vi "Find Center.vi"(7 "Tray Number":dbl format="%#_13g", 9 "XYZTheta":dbl[](array[numeric]), 10 "Motion.lvclass":refnum<class "Motion.lvclass">) -> (1 "XYZTheta Centers":dbl[][](array[numeric]), 2 "Motion Out":refnum<class "Motion.lvclass">)   [LabVIEW 2016, in "Assembly Tray.lvclass"]
uses:
  Assembly Tray.lvclass
  Find Tray.ctl
  Controller/Motion/Motion.lvclass
  Controller/Camera/Machine Vision.ctl
  Controller/Camera/Camera.lvclass
panel:
  in  "Machine Vision":T1=enum."Tray Fiducials"
  out "Right Fiducial":dbl[](array[numeric])
  out "Left Fiducial":dbl[](array[numeric])
  out "Gantry":dbl[](array[numeric])
  out "Sum":dbl[](array[numeric])
  out "Camera":dbl[](array[numeric])
  in  "Carrier Tray":T2
  out "Image":T3(plugin-control)
  out "Center":dbl[](array[numeric])
  in  "Position Number":i16
  in  "Go to Center":bool
  in  "Calculate":bool
  in  "Record Bottom":bool
  in  "Record Top":bool
  in  "Go to Bottom Fiducial":bool
  in  "Go to Top Fiducial":bool
  in  "Joystick":bool
  in  "Stop":bool
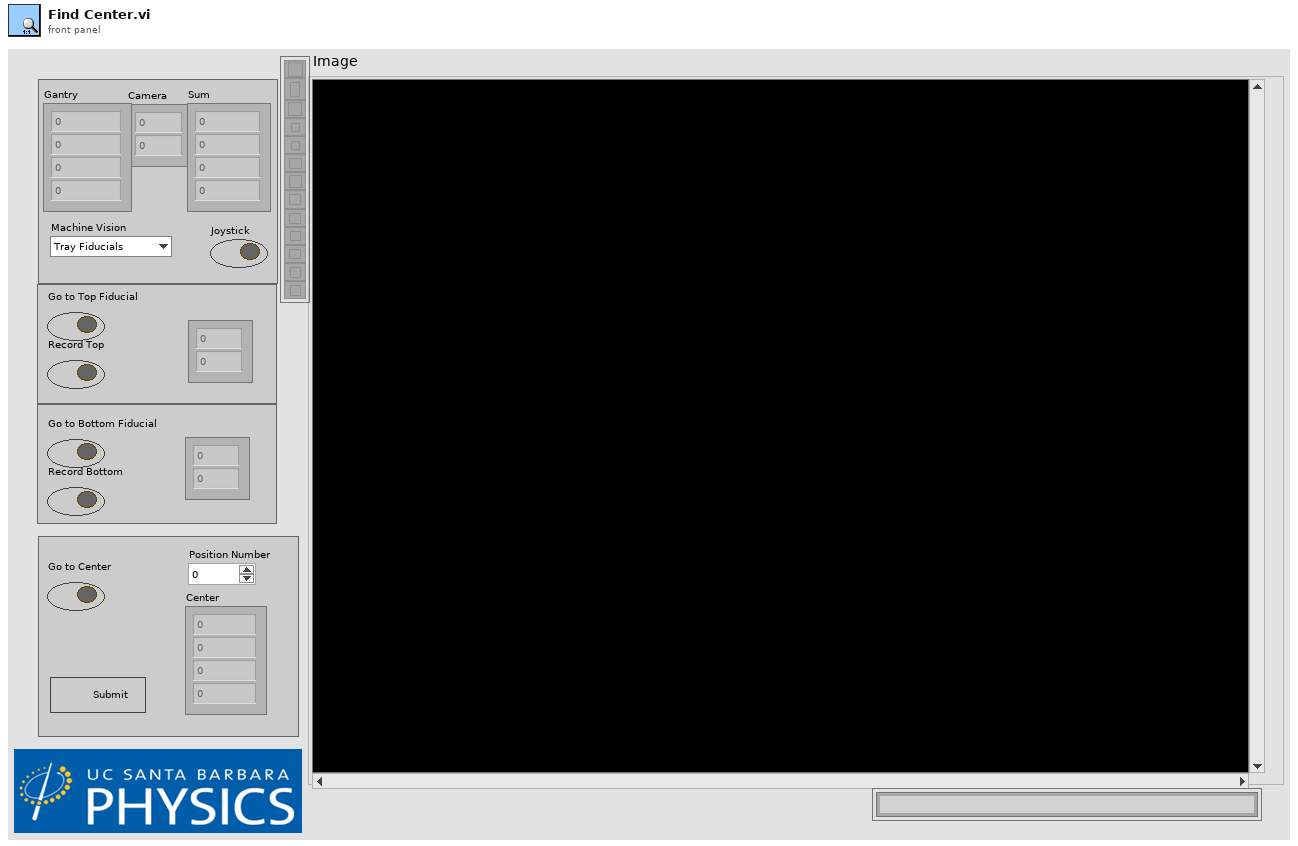
[diagram p1: front panel]
types:
  T1 = typedef "Camera.lvclass/Machine Vision.ctl" = enum16{"None", "Tray Fiducials", "HPK Silicon", "Hexaboard", "Corner (TL, BR)", "Corner (BL, TR)"}
  T2 = typedef "Assembly Tray.lvclass/Find Tray.ctl" = cluster{"Gantry Fiducials":dbl[], "Relative Coordinates":dbl[][], "Camera Fiducials":dbl[][], "XYZTheta Centers":dbl[][], "Workspace Center":dbl[], "Syringe Relative Coordinates":dbl[], "Gantry Region":dbl, "Fiducials":path}
  T3 = typedef "IMAQ Image.ctl" = refnum<image>
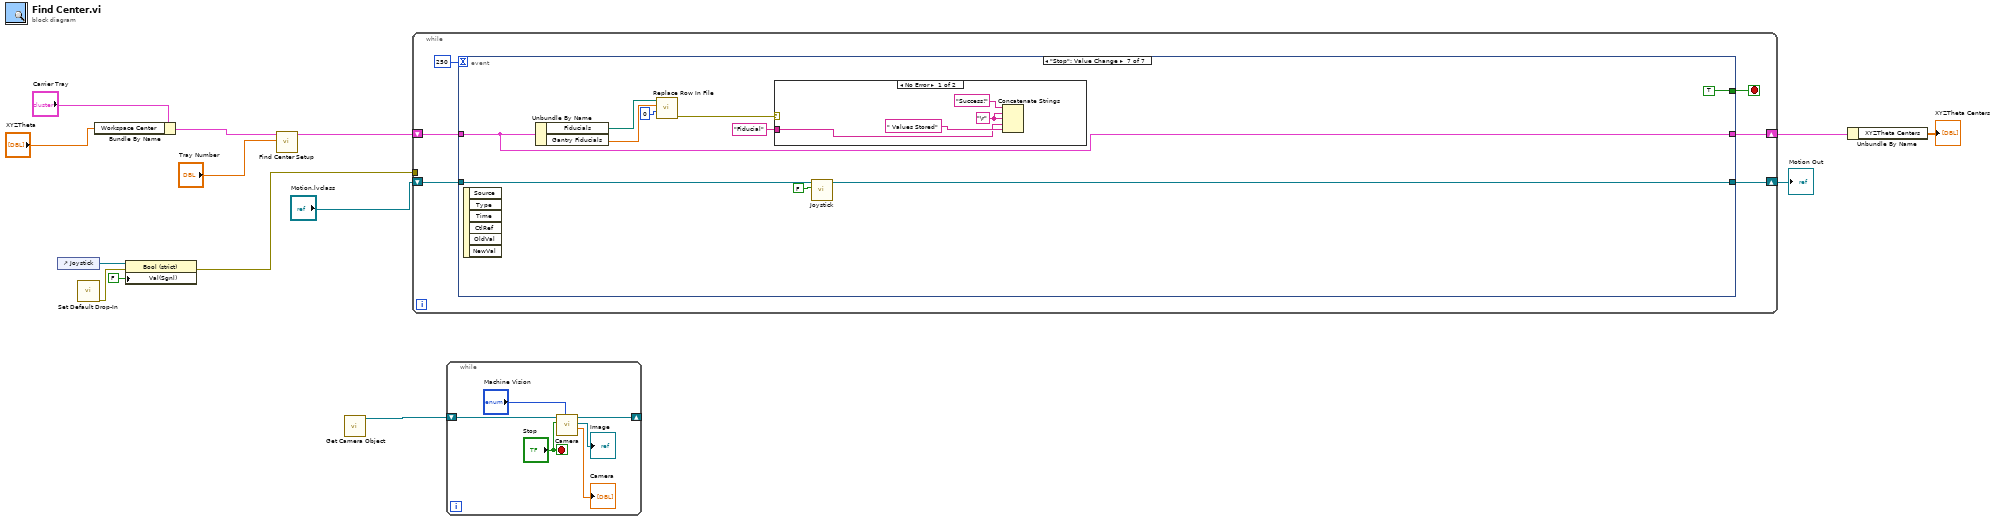
[diagram p0: block diagram]
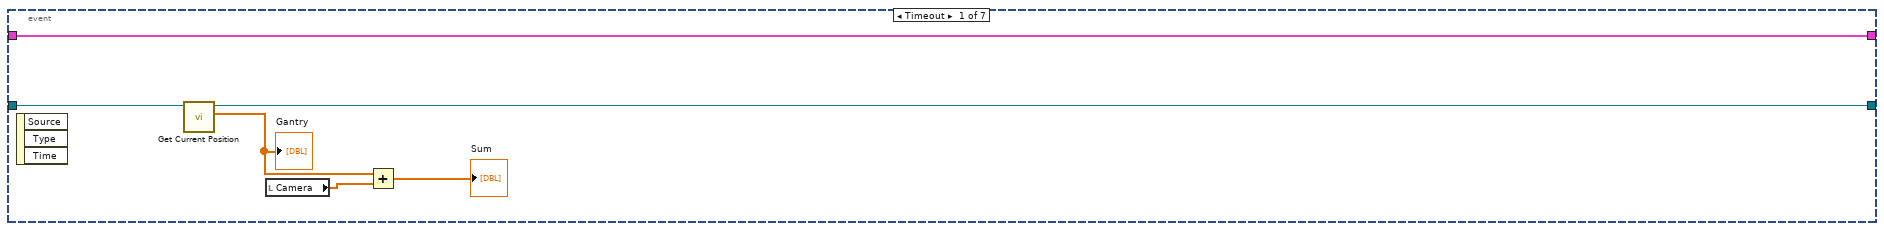
[diagram p2: hidden frame]
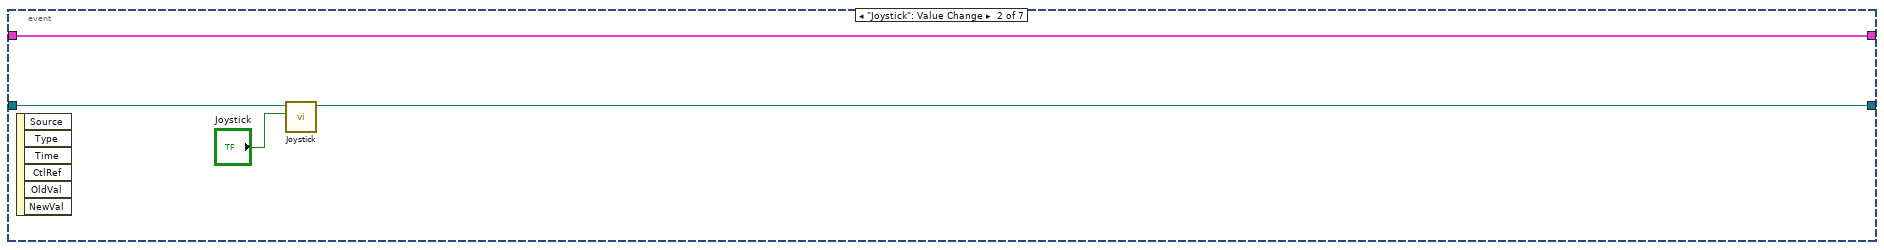
[diagram p3: hidden frame]
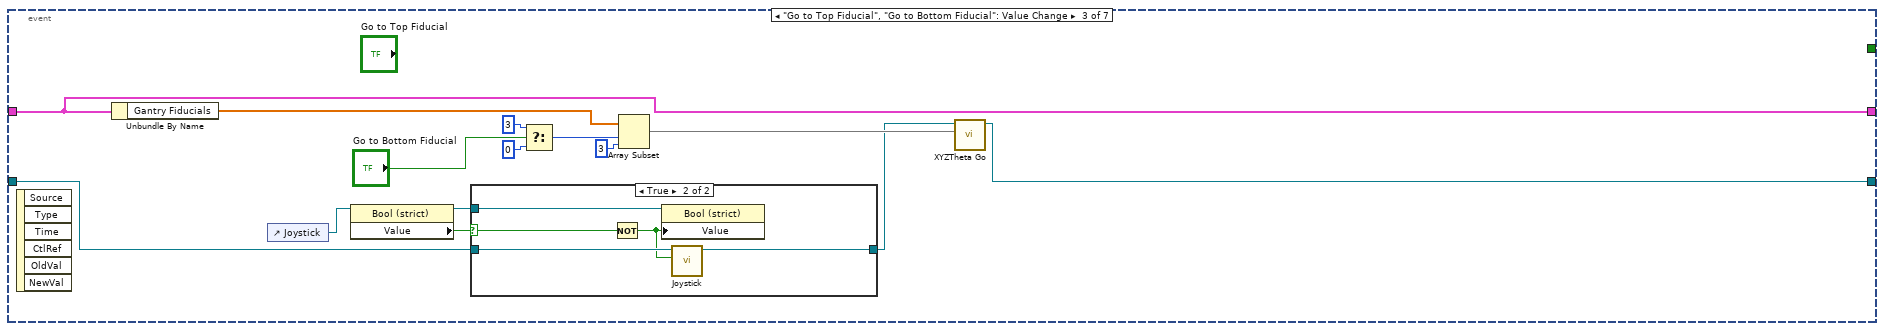
[diagram p4: hidden frame]
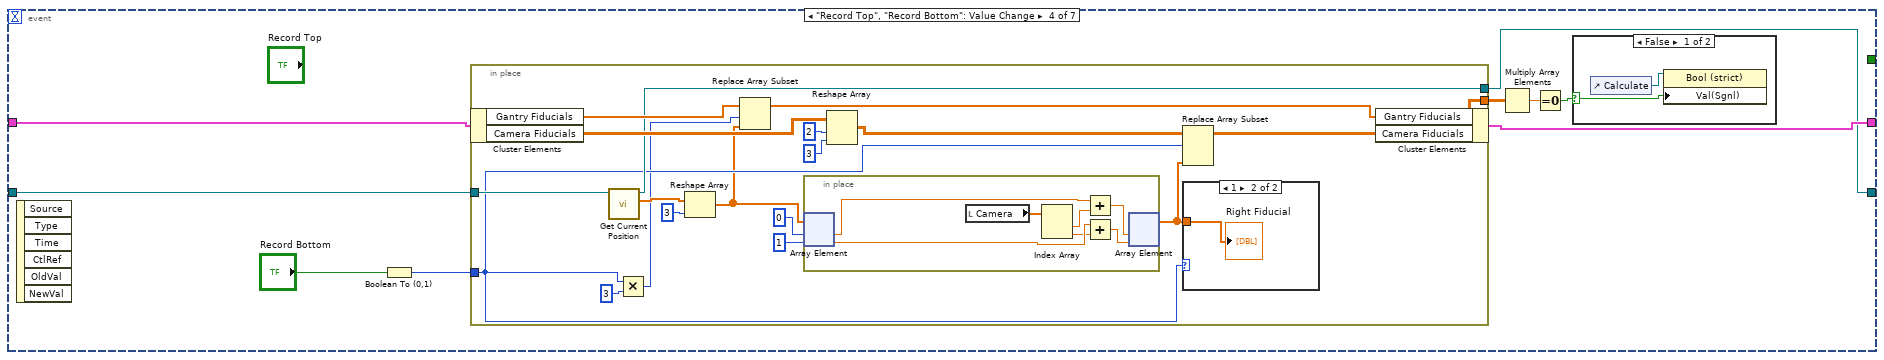
[diagram p6: hidden frame]
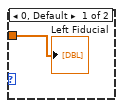
[diagram p8: hidden frame]
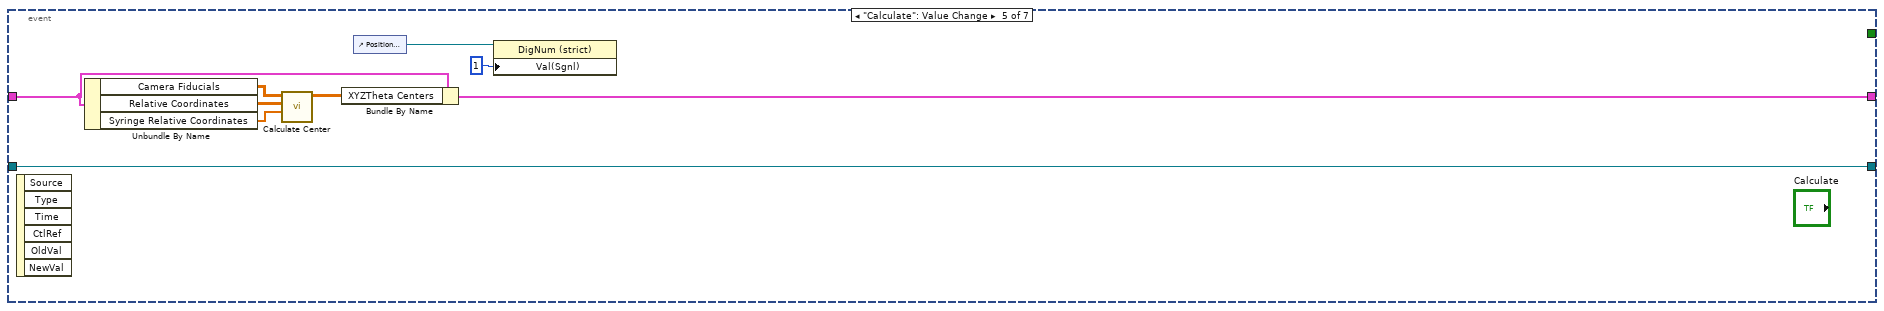
[diagram p9: hidden frame]
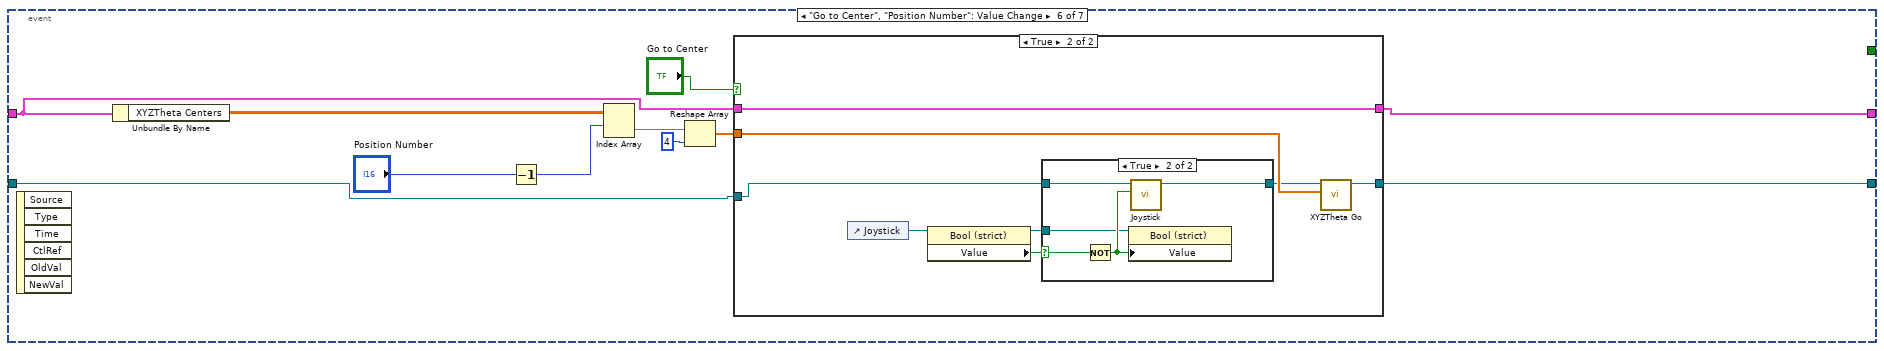
[diagram p10: hidden frame]
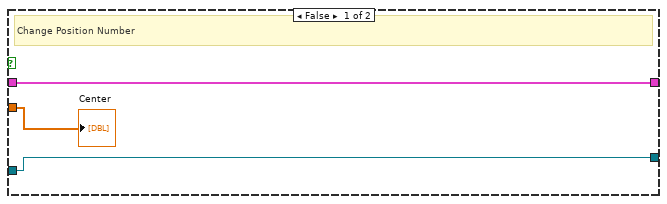
[diagram p11: hidden frame]
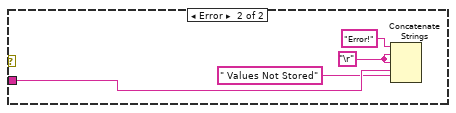
[diagram p13: hidden frame]
diagram:
  n1 = control-ref of="Joystick"() -> (w14:refnum<vi>)
  n2 = call "Set Default Drop-In.vi"() -> ("error out"=w6:errorcluster)  [unwired: 11 in]
  n3 = Bundle By Name(cluster="Carrier Tray", "Workspace Center"="XYZTheta") -> (w8:T2)
  n4 = property class="Bool (strict)"(reference=w14, error in=w6, "Val(Sgnl)"=FALSE) -> (error out=w12:errorcluster)  [unwired: 1 out]
  n5 = call "Find Center Setup.vi"("Carrier Tray"=w8, "Tray Number"="Tray Number") -> ("Assembly Tray Out"=w11:T2)  [unwired: 8 in]
  n6 = call "Get Camera Object.vi"() -> ("Camera out"=w1:refnum<class "Camera.lvclass">)  [unwired: 10 in, 1 out]
  n7 = while {
    shift-right: [w19] -> w10
    shift-left: w11 -> [w20]
    tunnel: w12 -> [_]
    shift-right: [w15] -> w3
    shift-left: "Motion.lvclass" -> [w16]
    stop <- w18 stop-if-true
    n8 = event shown="[6] \"Stop\": Value Change" {
      selector: _ -> [_ _ _ _ _ _ _]
      dyn-events: _ -> [_ _ _ _ _ _ _]
      timeout: 250 -> [_ _ _ _ _ _ _]
      tunnel: [w22 w28 w44 w59 w91 w104 w129] -> w19
      tunnel: w20 -> [w22 w28 w44 w53 w95 w105 w129]
      tunnel: [_ _ _ _ _ _ TRUE] -> w18
      tunnel: w16 -> [w23 w29 w33 w52 w89 w102 w131]
      tunnel: [w21 w27 w43 w51 w89 w101 w130] -> w15
      event Timeout {
        n9 = event-data() -> ()  [unwired: 1 in, 3 out]
        n10 = call-dynamic "Get Current Position.vi"("Motion in"=w23) -> ("XYZTheta Out"=w24:dbl[], "Motion out"=w21:refnum<class "Motion.lvclass">)  [unwired: 8 in, 1 out]
        "Gantry" <- w24
        n11 = local read "Camera"() -> (w26:dbl[])
        n12 = Add(x=w24, y=w26) -> (x+y=→"Sum":dbl[])
      }
      event "Joystick": Value Change {
        n13 = event-data() -> ()  [unwired: 1 in, 6 out]
        n14 = call-dynamic "Joystick.vi"("Joystick"="Joystick", "Motion in"=w29) -> ("Motion out"=w27:refnum<class "Motion.lvclass">)  [unwired: 8 in, 1 out]
      }
      event "Go to Top Fiducial", "Go to Bottom Fiducial": Value Change {
        n15 = event-data() -> ()  [unwired: 1 in, 6 out]
        n16 = Unbundle By Name(w44) -> ("Gantry Fiducials"=w41:dbl[])
        n17 = control-ref of="Joystick"() -> (w42:refnum<vi>)
        n18 = property class="Bool (strict)"(reference=w42) -> (reference out=w31:refnum<vi>, "Value"=w34:bool)  [unwired: 1 in, 1 out]
        n19 = case shown="True" w34 {
          selector: w34 -> [_ w50]
          tunnel: w33 -> [w45 w49]
          tunnel: [w45 w48] -> w32
          tunnel: w31 -> [_ w46]
          frame False {
          }
          frame True {
            n20 = Not(x=w50) -> (.not. x?=w47:bool)
            n21 = property class="Bool (strict)"(reference=w46, "Value"=w47) -> ()  [unwired: 1 in, 2 out]
            n22 = call-dynamic "Joystick.vi"("Joystick"=w47, "Motion in"=w49) -> ("Motion out"=w48:refnum<class "Motion.lvclass">)  [unwired: 8 in, 1 out]
          }
        }
        n23 = Select(t=3, s="Go to Bottom Fiducial", f=0) -> (s? t:f=w39:i32)
        n24 = Array Subset(array=w41, index=w39, length=3) -> (w35:dbl[])
        n25 = call "XYZTheta Go.vi"("XYZTheta In"=w35, "Motion in"=w32) -> ("Motion out"=w43:refnum<class "Motion.lvclass">)  [unwired: 7 in, 2 out]
      }
      event "Record Top", "Record Bottom": Value Change {
        n26 = event-data() -> ()  [unwired: 1 in, 6 out]
        n27 = Boolean To (0,1)(Boolean="Record Bottom") -> (0, 1=w55:i16)
        n28 = in-place {
          in-place-border: [w73] -> w56
          in-place-border: w55 -> [w66]
          in-place-border: w52 -> [w68]
          in-place-border: [w67] -> w51
          n29 = in-place-cluster #1(w53) -> ("Gantry Fiducials"=w70:dbl[], "Camera Fiducials"=w77:dbl[][])
          n30 = call-dynamic "Get Current Position.vi"("Motion in"=w68) -> ("XYZTheta Out"=w71:dbl[], "Motion out"=w67:refnum<class "Motion.lvclass">)  [unwired: 8 in, 1 out]
          n31 = Multiply(x=w66, y=i16 3) -> (x*y=w64:i16)
          n32 = Reshape Array(w71, 3 ("dimension size")) -> (w63:dbl[])
          n33 = Replace Array Subset(array=w70, new element=w63, index=w64) -> (w69:dbl[])
          n34 = in-place {
            n35 = in-place-array #2(w63, 0, 1) -> (w85:dbl, w83:dbl)
            n36 = local read "Camera"() -> (w86:dbl[])
            n37 = Index Array(array=w86) -> (element #1=w84:dbl, element #2=w82:dbl)  [unwired: 2 in]
            n38 = Add(x=w85, y=w84) -> (x+y=w80:dbl)
            n39 = Add(x=w83, y=w82) -> (x+y=w81:dbl)
            n40 = in-place-array #2(w80, w81) -> (w62:dbl[])  [unwired: 2 out]
          }
          n41 = Reshape Array(w77, 2 ("length"), 3 ("dimension size")) -> (w76:dbl[][])
          n42 = Replace Array Subset(array=w76, new element=w62, index (row)=w66) -> (w73:dbl[][])  [unwired: 1 in]
          n43 = case shown="1" w66 {
            tunnel: w62 -> [w87 w88]
            frame 0, Default {
              "Left Fiducial" <- w87
            }
            frame 1 {
              "Right Fiducial" <- w88
            }
          }
          n44 = in-place-cluster #1("Gantry Fiducials"=w69, "Camera Fiducials"=w73) -> (w59:T2)
        }
        n45 = Multiply Array Elements(1:w56) -> (0:w58:dbl)
        n46 = Equal To 0?(x=w58) -> (x = 0?=w57:bool)
        n47 = case shown="False" w57 {
          selector: w57 -> [w60 _]
          frame False {
            n48 = control-ref of="Calculate"() -> (w61:refnum<vi>)
            n49 = property class="Bool (strict)"(reference=w61, "Val(Sgnl)"=w60) -> ()  [unwired: 1 in, 2 out]
          }
          frame True {
          }
        }
      }
      event "Calculate": Value Change {
        n50 = event-data() -> ()  [unwired: 1 in, 6 out]
        n51 = Unbundle By Name(w95) -> ("Camera Fiducials"=w94:dbl[][], "Relative Coordinates"=w93:dbl[][], "Syringe Relative Coordinates"=w90:dbl[])
        n52 = call "Calculate Center.vi"("Syringe Coordinates"=w90, "Relative Coordinates"=w93, "Fiducial Measurements"=w94) -> ("XYZTheta Centers"=w92:dbl[][])  [unwired: 8 in]
        n53 = Bundle By Name(cluster=w95, "XYZTheta Centers"=w92) -> (w91:T2)
        n54 = control-ref of="Position Number"() -> (w97:refnum<vi>)
        n55 = property class="DigNum (strict)"(reference=w97, "Val(Sgnl)"=i16 1 ("Value (Signaling)")) -> ()  [unwired: 1 in, 2 out]
      }
      event "Go to Center", "Position Number": Value Change {
        n56 = event-data() -> ()  [unwired: 1 in, 6 out]
        n57 = Unbundle By Name(w105) -> ("XYZTheta Centers"=w108:dbl[][])
        n58 = Decrement(x="Position Number") -> (x-1=w106:i16)
        n59 = Index Array(array=w108, index (row)=w106) -> (element=w99:dbl[])  [unwired: 1 in]
        n60 = Reshape Array(w99, u32 4) -> (w98:dbl[])
        n61 = case shown="True" "Go to Center" {
          tunnel: w98 -> [w111 w117]
          tunnel: w105 -> [w110 w119]
          tunnel: [w110 w119] -> w104
          tunnel: w102 -> [w109 w113]
          tunnel: [w109 w118] -> w101
          frame False {
            # "Change Position Number"
            "Center" <- w111
          }
          frame True {
            n62 = control-ref of="Joystick"() -> (w116:refnum<vi>)
            n63 = property class="Bool (strict)"(reference=w116) -> (reference out=w114:refnum<vi>, "Value"=w115:bool)  [unwired: 1 in, 1 out]
            n64 = case shown="True" w115 {
              selector: w115 -> [_ w125]
              tunnel: w113 -> [w120 w124]
              tunnel: [w120 w123] -> w112
              tunnel: w114 -> [_ w121]
              frame False {
              }
              frame True {
                n65 = Not(x=w125) -> (.not. x?=w122:bool)
                n66 = property class="Bool (strict)"(reference=w121, "Value"=w122) -> ()  [unwired: 1 in, 2 out]
                n67 = call-dynamic "Joystick.vi"("Joystick"=w122, "Motion in"=w124) -> ("Motion out"=w123:refnum<class "Motion.lvclass">)  [unwired: 8 in, 1 out]
              }
            }
            n68 = call "XYZTheta Go.vi"("XYZTheta In"=w117, "Motion in"=w112) -> ("Motion out"=w118:refnum<class "Motion.lvclass">)  [unwired: 7 in, 2 out]
          }
        }
      }
      event "Stop": Value Change {
        n69 = event-data() -> ()  [unwired: 1 in, 6 out]
        n70 = Unbundle By Name(w129) -> ("Fiducials"=w127:path, "Gantry Fiducials"=w128:dbl[])
        n71 = call "Replace Row In File.vi"("Index"=0, "Insert Array"=w128, "Path"=w127) -> ("error out"=w134:errorcluster)  [unwired: 8 in]
        n72 = case shown="No Error" w134 {
          tunnel: "Fiducial" -> [w136 w143]
          frame No Error {
            w137 = "\r"
            n73 = Concatenate Strings("Success!", w137, w137, w136, " Values Stored") -> ()  [unwired: 1 out]
          }
          frame Error {
            w140 = "\r"
            n74 = Concatenate Strings("Error!", w140, w140, w143, " Values Not Stored") -> ()  [unwired: 1 out]
          }
        }
        n75 = call-dynamic "Joystick.vi"("Joystick"=FALSE, "Motion in"=w131) -> ("Motion out"=w130:refnum<class "Motion.lvclass">)  [unwired: 8 in, 1 out]
      }
    }
  }
  "Motion Out" <- w3
  n76 = while {
    shift-right: [w144] -> _
    shift-left: w1 -> [w149]
    stop <- "Stop" stop-if-true
    n77 = call "Camera.vi"("Machine Vision"="Machine Vision", "Stop"="Stop", "Camera in"=w149) -> ("Camera"=→"Camera":dbl[], "Image"=→"Image":T3, "Camera out"=w144:refnum<class "Camera.lvclass">)  [unwired: 5 in, 1 out]
  }
  n78 = Unbundle By Name(w10) -> ("XYZTheta Centers"=→"XYZTheta Centers":dbl[][])
